vi "goToStandby.vi"(8 "error in (no error)":errorcluster, 10 "model":refnum<class "Model.lvclass">, 11 "EnabledState in":refnum<class "EnabledState.lvclass">) -> (0 "error out":errorcluster, 2 "model 2":refnum<class "Model.lvclass">, 3 "EnabledState out":refnum<class "EnabledState.lvclass">)   [LabVIEW 2012, in "EnabledState.lvclass"]
uses:
  EnabledState.lvclass
  Model/Model/Model.lvclass
  Typedefs/StateSelector.ctl
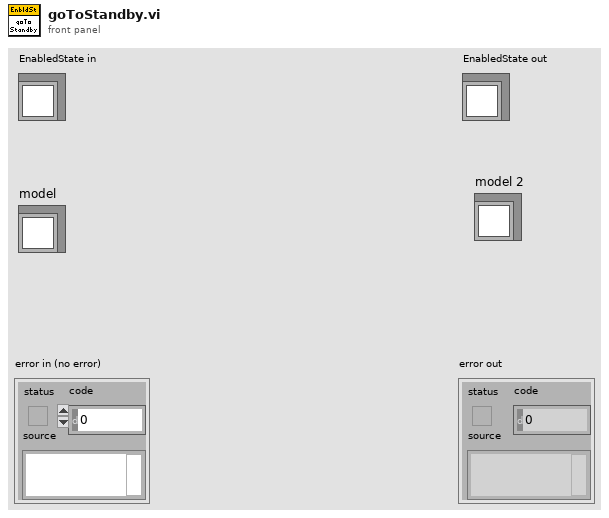
[diagram p1: front panel]
types:
  T1 = typedef "StateSelector.ctl" = enum16{"DataOnDemandState", "DataStreamingState", "FaultState", "OffState", "StandbyState"}
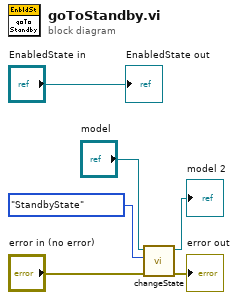
[diagram p0: block diagram]
diagram:
  n1 = call "changeState.vi"("error in (no error)"="error in (no error)", "State:"=StateSelector."StandbyState", "Model in"="model") -> ("error out"=→"error out":errorcluster, "Model out"=→"model 2":refnum<class "Model.lvclass">)  [unwired: 7 in]
  "EnabledState out" <- "EnabledState in"
